vi "getFrontEndPath.vi"(8 "error in (no error)":errorcluster, 11 "WinX32Settings in":refnum<class "WinX32Settings.lvclass">) -> (0 "error out":errorcluster, 2 "Path":path, 3 "WinX32Settings out":refnum<class "WinX32Settings.lvclass">)   [LabVIEW 2011, in "Tools.lvlib" / "Settings.lvlib" / "WinX32Settings.lvclass"]
uses:
  WinX32Settings.lvclass
  Filing/FileSystem/FileSystem.lvclass
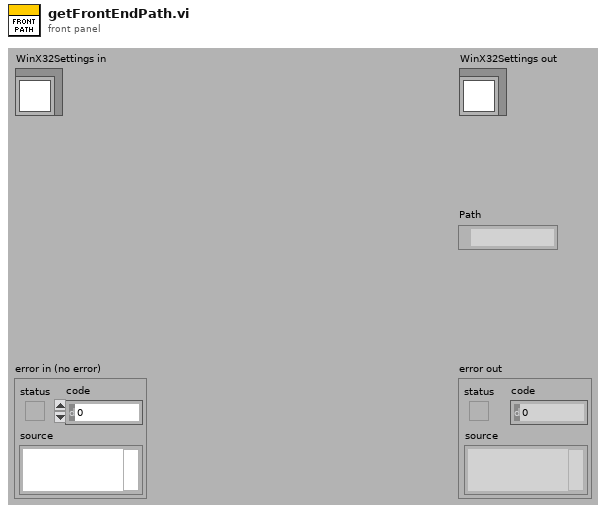
[diagram p1: front panel]
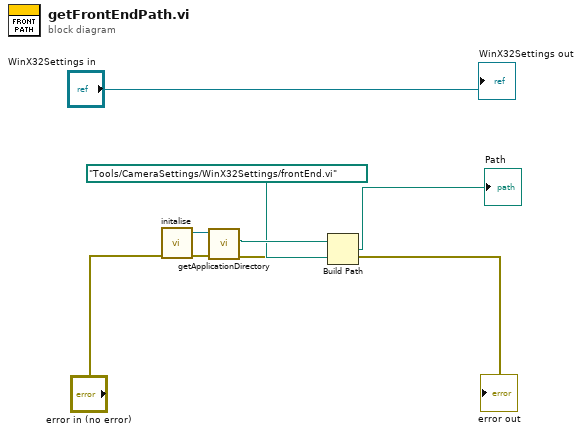
[diagram p0: block diagram]
diagram:
  n1 = call "initalise.vi"("error in (no error)"="error in (no error)") -> ("error out"=w7:errorcluster, "FileSystem out"=w8:refnum<class "FileSystem.lvclass">)  [unwired: 9 in]
  n2 = call-dynamic "getApplicationDirectory.vi"("error in (no error)"=w7, "FileSystem.lvclass in"=w8) -> ("error out"=→"error out":errorcluster, "ApplicationDirectory"=w6:path)  [unwired: 7 in, 1 out]
  n3 = Build Path(base path=w6, name or relative path=path "Tools/CameraSettings/WinX32Settings/frontEnd.vi") -> (appended path=→"Path":path)
  "WinX32Settings out" <- "WinX32Settings in"
